vi "Sort VI Ref Type.vi"(10 "Panel B":refnum<class "Panel.lvclass">, 11 "Panel A":refnum<class "Panel.lvclass">) -> (3 "Order":i32)   [LabVIEW 2018, in "OOPanel.lvlib"]
uses:
  OOPanel.lvlib
  Panel/Panel.lvclass
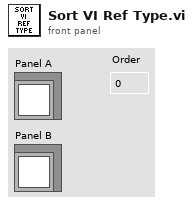
[diagram p1: front panel]
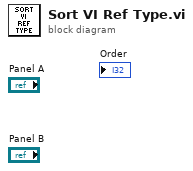
[diagram p0: block diagram]
diagram:
